vi "TrapezoidalMotionProfile.vi"(6 "Initialize":bool, 7 "dt":dbl, 10 "Time":dbl, 11 "Config":T2={"TargetPos"=10.0, "InitalPos"=0.0, "FinalVel"=0.0, "IntitialVel"=0.0, "MaxVel"=10.0, "MaxAccel"=10.0}) -> (0 "Done":bool, 2 "Velocity":dbl, 3 "Distance":dbl)   [LabVIEW 2017]
panel:
  out "AllData":T1
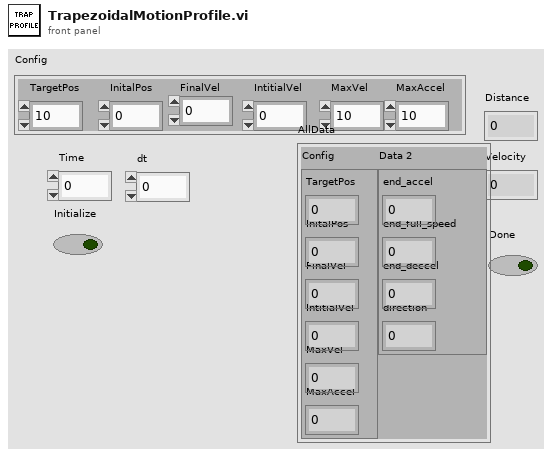
[diagram p1: front panel]
types:
  T1 = cluster{"Config":cluster{"TargetPos":dbl, "InitalPos":dbl, "FinalVel":dbl, "IntitialVel":dbl, "MaxVel":dbl, "MaxAccel":dbl}, "Data 2":cluster{"end_accel":dbl, "end_full_speed":dbl, "end_deccel":dbl, "direction":dbl}}
  T2 = cluster{"TargetPos":dbl, "InitalPos":dbl, "FinalVel":dbl, "IntitialVel":dbl, "MaxVel":dbl, "MaxAccel":dbl}
  T3 = cluster{"end_accel":dbl, "end_full_speed":dbl, "end_deccel":dbl, "direction":dbl}
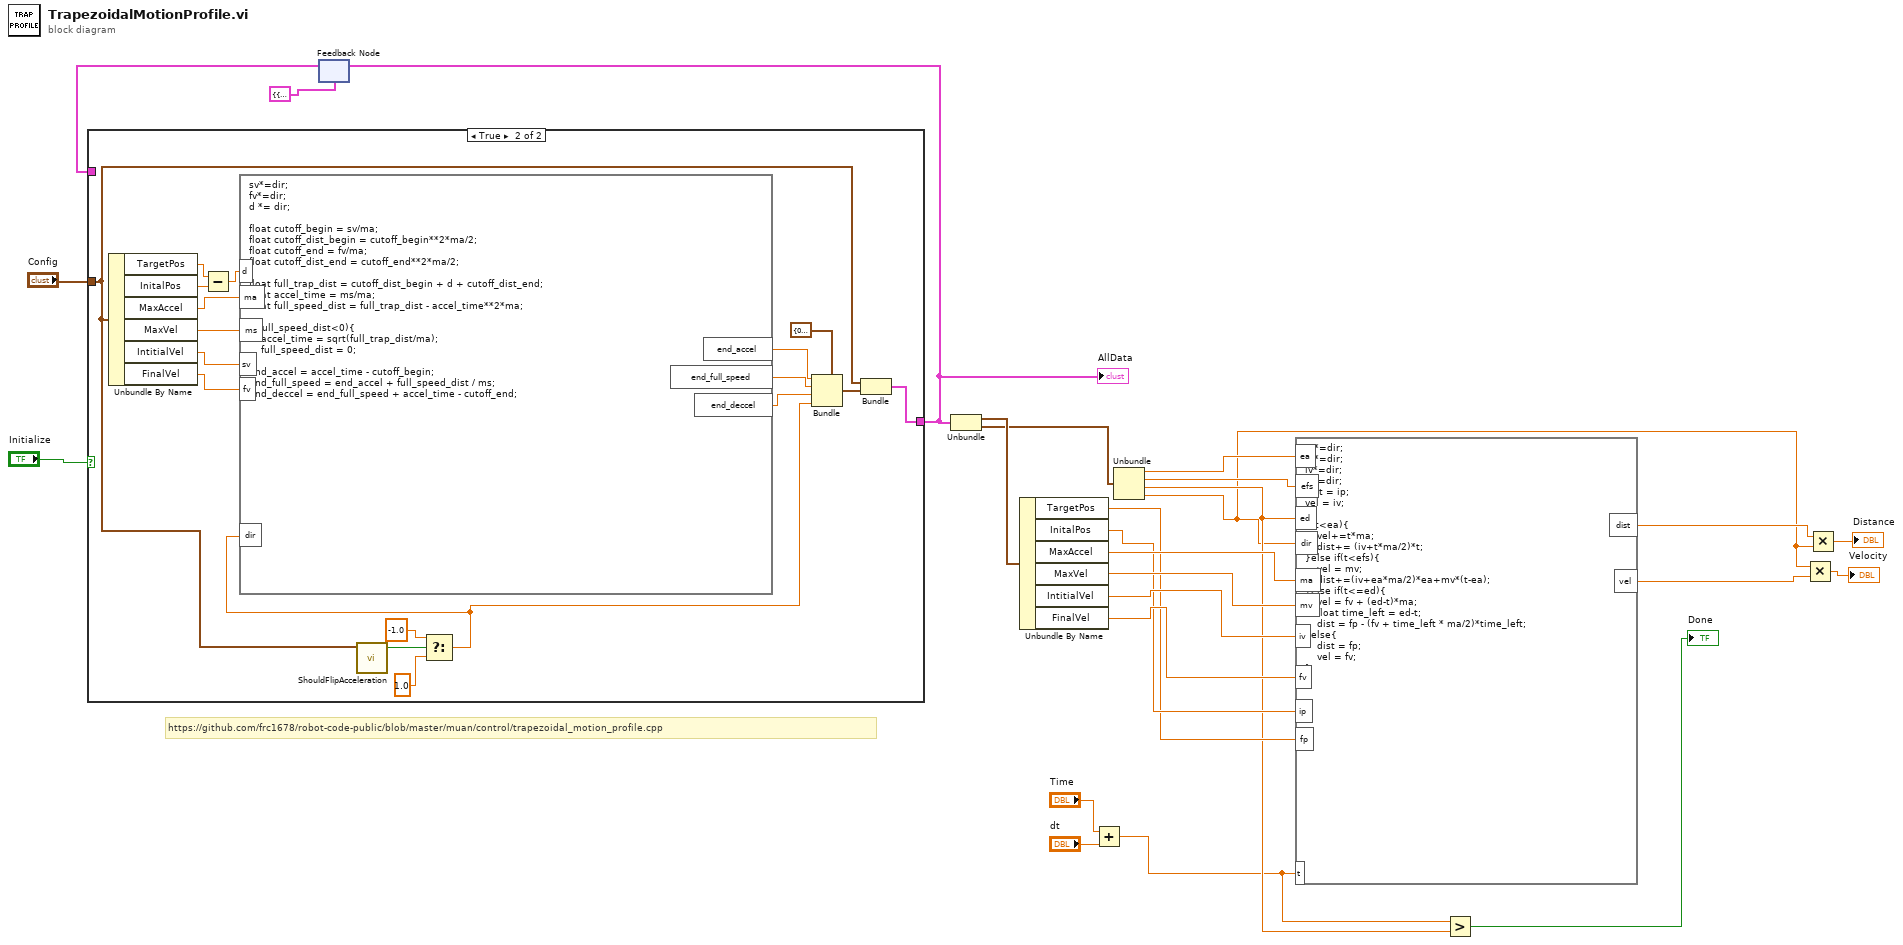
[diagram p0: block diagram]
diagram:
  # "https://github.com/frc1678/robot-code-public/blob/master/muan/control/trapezoidal_motion_profile.cpp"
  n1 = feedback #1(T1 {"Config"={"TargetPos"=10.0, "InitalPos"=0.0, "FinalVel"=0.0, "IntitialVel"=0.0, "MaxVel"=10.0, "MaxAccel"=10.0}, "Data 2"={"end_accel"=0.0, "end_full_speed"=0.0, "end_deccel"=0.0, "direction"=0.0}} ("AllData")) -> (w23:T1)
  n2 = case shown="True" "Initialize" {
    tunnel: "Config" -> [_ w37]
    tunnel: [w26 w27] -> w9
    tunnel: w23 -> [w26 _]
    frame False {
    }
    frame True {
      n3 = Unbundle By Name(w37) -> ("TargetPos"=w38:dbl, "InitalPos"=w39:dbl, "MaxAccel"=w44:dbl, "MaxVel"=w43:dbl, "IntitialVel"=w41:dbl, "FinalVel"=w40:dbl)
      n4 = Subtract(x=w38, y=w39) -> (x-y=w42:dbl)
      n5 = call "ShouldFlipAcceleration.vi"("Config"=w37) -> ("Flip?"=w33:bool)  [unwired: 10 in]
      n6 = Select(t=-1.0, s=w33, f=1.0) -> (s? t:f=w28:dbl)
      n7 = formula code="sv*=dir;\nfv*=dir;\nd *= dir;\n\nfloat cutoff_begin = sv/ma;\nfloat cutoff_dist_begin = cutoff_begin**2*ma/2;\nfloat cutoff_end = fv/ma;\nfloat cutoff_dist_end = cutoff_end**2*ma/2;\n\nfloat full_trap_dist = cutoff_dist_begin + d + cutoff_dist_end;\nfloat accel_time = ms/ma;\nfloat full_speed_dist = full_trap_dist - accel_time**2*ma;\n\nif(full_speed_dist<0){\n    accel_time = sqrt(full_trap_dist/ma);\n    full_speed_dist = 0;\n}\nend_accel = accel_time - cutoff_begin;\nend_full_speed = end_accel + full_speed_dist / ms;\nend_deccel = end_full_speed + accel_time - cutoff_end;"("ma"=w44, "ms"=w43, "d"=w42, "sv"=w41, "fv"=w40, "dir"=w28) -> ("end_accel"=w35:dbl, "end_full_speed"=w30:dbl, "end_deccel"=w29:dbl)
      n8 = Bundle(cluster=T3 {"end_accel"=0.0, "end_full_speed"=0.0, "end_deccel"=0.0, "direction"=0.0} ("Data 2"), "end_accel"=w35, "end_full_speed"=w30, "end_deccel"=w29, "direction"=w28) -> (w36:T3)
      n9 = Bundle("Config"=w37, "Data 2"=w36) -> (w27:T1)  [unwired: 1 in]
    }
  }
  "AllData" <- w9
  n10 = feedback-in #1(w9) -> ()
  n11 = Unbundle(w9) -> ("Config"=w8:T2, "Data 2"=w7:T3)
  n12 = Unbundle By Name(w8) -> ("TargetPos"=w16:dbl, "InitalPos"=w17:dbl, "MaxAccel"=w21:dbl, "MaxVel"=w20:dbl, "IntitialVel"=w19:dbl, "FinalVel"=w18:dbl)
  n13 = Add(x="Time", y="dt") -> (x+y=w4:dbl)
  n14 = Unbundle(w7) -> ("end_accel"=w15:dbl, "end_full_speed"=w14:dbl, "end_deccel"=w13:dbl, "direction"=w10:dbl)
  n15 = formula code="ip*=dir;\nfp*=dir;\niv*=dir;\nfv*=dir;\ndist = ip;\nvel = iv;\n\nif(t<ea){\n    vel+=t*ma;\n    dist+= (iv+t*ma/2)*t;\n}else if(t<efs){\n    vel = mv;\n    dist+=(iv+ea*ma/2)*ea+mv*(t-ea);\n}else if(t<=ed){\n    vel = fv + (ed-t)*ma;\n    float time_left = ed-t;\n    dist = fp - (fv + time_left * ma/2)*time_left;\n}else{\n    dist = fp;\n    vel = fv;\n}"("t"=w4, "ea"=w15, "efs"=w14, "ed"=w13, "ma"=w21, "iv"=w19, "mv"=w20, "fv"=w18, "ip"=w17, "fp"=w16, "dir"=w10) -> ("dist"=w12:dbl, "vel"=w11:dbl)
  n16 = Greater?(x=w4, y=w13) -> (0:→"Done":bool)
  n17 = Multiply(x=w10, y=w11) -> (x*y=→"Velocity":dbl)
  n18 = Multiply(x=w12, y=w10) -> (x*y=→"Distance":dbl)
